vi "User event LV2.vi"(0 "Event data":T1, 11 "Error in":errorcluster, 13 "Operation":T2) -> (4 "Event data ref":refnum<user-event>, 15 "Error out":errorcluster)   [LabVIEW 2020, in "PSRR Monitor.lvlib"]
doc: "This SubVI is used as user event LV2 which is used for creating, generating and getting reference of user events which are created."
uses:
  PSRR Monitor.lvlib
  Typedefs/User LV2 operations.ctl
  Typedefs/User LV2 data.ctl
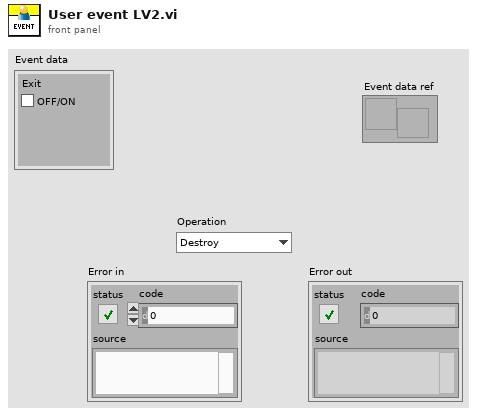
[diagram p1: front panel]
types:
  T1 = typedef "PSRR Monitor.lvlib/User LV2 data.ctl" = cluster{"Exit":bool}
  T2 = typedef "PSRR Monitor.lvlib/User LV2 operations.ctl" = enum16{"Destroy", "Get ref", "Generate", "Create"}
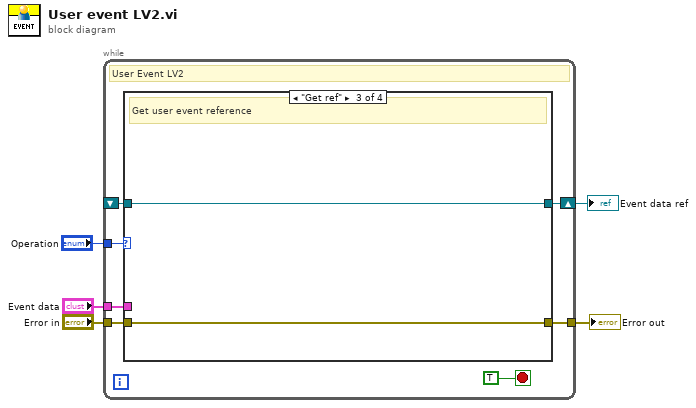
[diagram p0: block diagram]
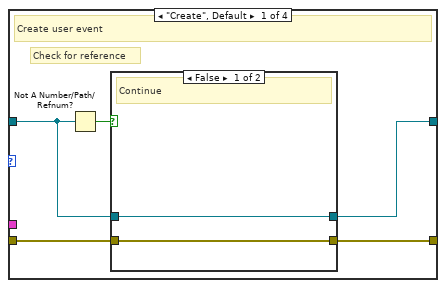
[diagram p2: hidden frame]
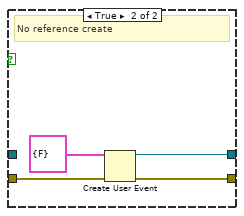
[diagram p3: hidden frame]
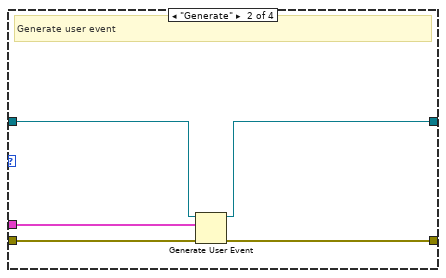
[diagram p4: hidden frame]
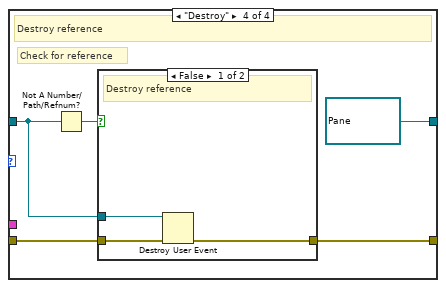
[diagram p5: hidden frame]
diagram:
  n1 = while {
    tunnel: "Error in" -> [w10]
    tunnel: "Operation" -> [w12]
    shift-right: [w8] -> w1
    shift-left: _ -> [w7]
    tunnel: [w9] -> w3
    tunnel: "Event data" -> [w6]
    stop <- TRUE stop-if-true
    # "User Event LV2"
    n2 = case shown="\"Get ref\"" w12 {
      tunnel: w10 -> [w16 w28 w29 w35]
      tunnel: [w15 w27 w29 w34] -> w9
      tunnel: [w14 w24 w30 refnum<user-event> refnum ("Event data")] -> w8
      tunnel: w7 -> [w13 w25 w30 w32]
      tunnel: w6 -> [_ w26 _ _]
      frame "Create", Default {
        # "Check for reference"
        # "Create user event"
        n3 = Not A Number/Path/Refnum?(number/path/refnum=w13) -> (NaN/Path/Refnum?=w17:bool)
        n4 = case shown="False" w17 {
          tunnel: w16 -> [w19 w23]
          tunnel: [w19 w22] -> w15
          tunnel: [w18 w20] -> w14
          tunnel: w13 -> [w18 _]
          frame False {
            # "Continue"
          }
          frame True {
            # "No reference create"
            n5 = Create User Event(user event datatype=T1 {"Exit"=FALSE} ("Event data"), error in=w23) -> (user event=w20:refnum<user-event>, error out=w22:errorcluster)
          }
        }
      }
      frame "Generate" {
        # "Generate user event"
        n6 = Generate User Event(user event=w25, event data cluster=w26, error in=w28) -> (user event out=w24:refnum<user-event>, error out=w27:errorcluster)  [unwired: 1 in]
      }
      frame "Get ref" {
        # "Get user event reference"
      }
      frame "Destroy" {
        # "Check for reference"
        # "Destroy reference"
        n7 = Not A Number/Path/Refnum?(number/path/refnum=w32) -> (NaN/Path/Refnum?=w33:bool)
        n8 = case shown="False" w33 {
          tunnel: w35 -> [w38 w39]
          tunnel: [w37 w39] -> w34
          tunnel: w32 -> [w36 _]
          frame False {
            # "Destroy reference"
            n9 = Destroy User Event(user event=w36, error in=w38) -> (error out=w37:errorcluster)
          }
          frame True {
            # "Do not destroy if no reference is present"
          }
        }
      }
    }
  }
  "Error out" <- w3
  "Event data ref" <- w1
